vi "FPGA_main.vi"() -> ()   [LabVIEW 2020]
uses:
  <vilib>/rvi/Emulation/niFpgaGetClockAttributes.vi
  <vilib>/rvi/Emulation/niFpgaSctlEmulationGetInTimedLoop.vi
  <vilib>/rvi/Emulation/niFpgaEmulationReportErrorSimple.vi
  <vilib>/rvi/eio/common/nirviEmuTemplateMethod_errors.vi
  <vilib>/rvi/Emulation/niFpgaCriticalErrorInLSC.vi
  <vilib>/eio/EIONode/EIONode.xnode
panel:
  out "AO loop time [ticks]":u32
  out "AI loop time [ticks]":u32
  out "C_AI1_readValue":i16
  out "C_AI0_readValue":i16
  in  "C_AO0_writeValue":i16
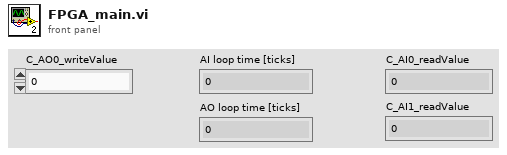
[diagram p1: front panel]
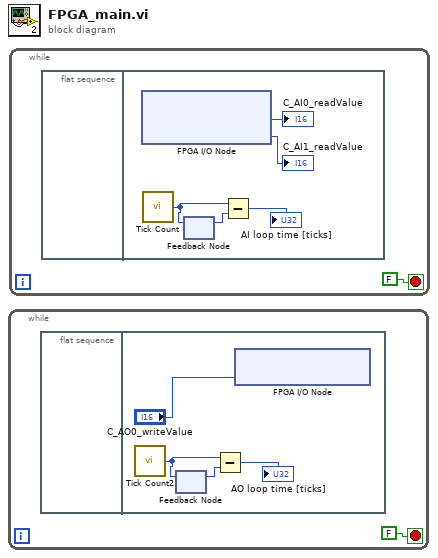
[diagram p0: block diagram]
diagram:
  n1 = while {
    stop <- FALSE stop-if-true
    n2 = flat-sequence {
      frame #0 {
      }
      frame #1 {
        n3 = call "Tick Count2"() -> ("Tick Count(Ticks)"=w2:u32)
        n4 = feedback #1() -> (w3:u32)  [unwired: 1 in]
        n5 = feedback-in #1(w2) -> ()
        n6 = Subtract(x=w2, y=w3) -> (x-y=→"AO loop time [ticks]":u32)
        n7 = xnode "FPGA I/O Node"("ConnectorC/AO0"="C_AO0_writeValue") -> ()  [unwired: 1 in, 1 out]
      }
    }
  }
  n8 = while {
    stop <- FALSE stop-if-true
    n9 = flat-sequence {
      frame #0 {
      }
      frame #1 {
        n10 = xnode "FPGA I/O Node"() -> ("ConnectorC/AI0"=→"C_AI0_readValue":i16, "ConnectorC/AI1"=→"C_AI1_readValue":i16)  [unwired: 2 in, 2 out]
        n11 = call "Tick Count"() -> ("Tick Count(Ticks)"=w9:u32)
        n12 = feedback-in #2(w9) -> ()
        n13 = feedback #2() -> (w8:u32)  [unwired: 1 in]
        n14 = Subtract(x=w9, y=w8) -> (x-y=→"AI loop time [ticks]":u32)
      }
    }
  }
